vi "Launch AIP Actor.vi"(11 "RDS Root Actor in":refnum<class "RDS Root Actor.lvclass">) -> (3 "RDS Root Actor out":refnum<class "RDS Root Actor.lvclass">)   [LabVIEW 2015, in "RDS Root Actor.lvlib" / "RDS Root Actor.lvclass"]
uses:
  RDS Root Actor.lvclass
  AIP Instrument/AIP Instrument/AIP Instrument.lvclass
  Libraries/RDS Framework/RDS Message ID.ctl
  Libraries/RDS Instruments/RDS Instrument Enums.ctl
  RDS Parent Actor/RDS Parent Actor/RDS Parent Actor.lvclass/RDS Parent Actor.ctl
  RDS Serial Instrument Actor/RDS Serial Instrument Actor.lvclass/RDS Serial Instrument Actor.ctl
  RDS Parent Actor/RDS Parent Actor/RDS Parent Actor.lvclass
  Libraries/RDS Child Messages/RDS Child Messages.lvlib
  RDS Serial Instrument Actor/RDS Serial Instrument Actor.lvclass
  Libraries/Configuration Library/RDS Configuration Library.lvlib
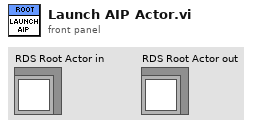
[diagram p1: front panel]
types:
  T1 = typedef "RDS Child Messages.lvlib/RDS Message ID.ctl" = enum16{"RDS Hello World", "String Message", "AIP_Status", "AIP_Command", "GPS_Data", "MCB_Command", "MCB_Status", "Compass_Data", "Depth_Data", "Battery_Data", "Contoller_State", "Set_Mag_Dev", "BTB_Shutdown", "State_Sample_Request", "State_Sample", "PID_Gains_Set", "Helm_Limiter_Set", "Helm_Heading_Command", "Helm_Steering_Command", "Helm_Status", "Controller_Message", "AIP_Set_Min_Depth", "Mission_Controller_State", "Mission_Upload", "Mission_Set_Op_and_Run", "Mission_Settings_Set"}
  T2 = typedef "RDS Configuration Library.lvlib/RDS Instrument Enums.ctl" = enum16{"AIP", "GPS", "Compass", "PORT Motor", "STBD Motor", "LSR", "Depth Transducer", "BTB"}
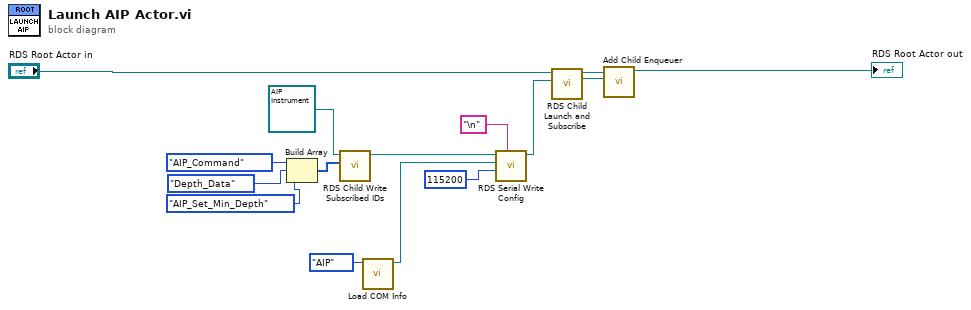
[diagram p0: block diagram]
diagram:
  n1 = Build Array(RDS_Message_ID."AIP_Command" ("RDS Message"), RDS_Message_ID."Depth_Data" ("RDS Message"), RDS_Message_ID."AIP_Set_Min_Depth" ("RDS Message")) -> (w8:T1[])
  n2 = call "RDS Child Write Subscribed IDs.vi"("Subscribed IDs"=w8, "RDS Parent Actor in"=refnum<class "AIP Instrument.lvclass"> refnum ("AIP Instrument.lvlib:AIP Instrument.lvclass")) -> ("RDS Parent Actor out"=w9:refnum<class "AIP Instrument.lvclass">)  [unwired: 8 in, 1 out]
  n3 = call "Load COM Info.vi"("Serial Instrument"=RDS_Instrument_Enums."AIP") -> ("COM Port"=w3:refnum<visa-resource-name>)  [unwired: 10 in]
  n4 = call "RDS Serial Write Config.vi"("Termination Char(s)"="\n", "baud rate"=u32 115200, "VISA resource name"=w3, "RDS Serial Instrument Actor in"=w9) -> ("RDS Serial Instrument Actor out"=w11:refnum<class "AIP Instrument.lvclass">)  [unwired: 6 in, 1 out]
  n5 = call "RDS Child Launch and Subscribe.vi"("RDS Child in"=w11, "Caller Actor in"="RDS Root Actor in") -> ("Nested Actor's Enqueuer"=w14:refnum<class "Message Enqueuer.lvclass">, "Caller Actor Out"=w13:refnum<class "RDS Root Actor.lvclass">)  [unwired: 7 in, 1 out]
  n6 = call "Add Child Enqueuer.vi"("Nested Actor's Enqueuer"=w14, "RDS Root Actor in"=w13) -> ("RDS Root Actor out"=→"RDS Root Actor out":refnum<class "RDS Root Actor.lvclass">)  [unwired: 8 in, 1 out]
